vi "Autonomous Independent.vi"   [LabVIEW 2017]
doc: "This VI is called when autonomous begins, and will automatically be terminated when autonomous ends. You can carry out timed or sensor driven robot movement independently without needing to return to the caller."
uses:
  <vilib>/Rock Robotics/WPI/SafetyOutput/WPI_SafetyOutputConfigMenu.ctl
  <vilib>/Rock Robotics/Network Tables/NT Read String.vi
  <vilib>/Rock Robotics/Network Tables/NT Read Number.vi
  <vilib>/Rock Robotics/WPI/Utilities/WPI_GetSetVariantRefNum.vi
  <vilib>/Rock Robotics/WPI/RobotDrive/WPI_RobotDriveArcadeDrive_Standard(NoSaturation).vi
panel:
  # "Be sure to right-click and choose Data Operations>>Make Current Value default if you want to save the array values with the VI"
types:
  T1 = typedef "WPI_SafetyOutputConfigMenu.ctl" = enum16{"Enable", "Disable"}
  T2 = typedef "WPI_RobotDriveDevRef.ctl" = cluster{"DevStatus":errorcluster, "Motors[]":T3[], "Square Inputs":bool, "Max Output":dbl}
  T3 = typedef "WPI_MotorControlDeviceRef.ctl" = cluster{"DeviceStatus":errorcluster, "Type":T4, "PWM":cluster{"PWM Channel":T5, "DeadBand":T6}, "CAN":cluster{"Device Number":u8, "SetOutput VI Ref":variant, "GetOutput VI Ref":variant, "Enable VI Ref":variant, "Disable VI Ref":variant, "Data":variant}, "Invert":bool, "DIO PWM":cluster{"PWM \"Enable\" Channel":T5, "DIOChannel":T7, "PWM Rate":dbl}}
  T4 = typedef "WPI_MotorControlType.ctl" = enum16{"PWM", "CAN", "DIO PWM"}
  T5 = typedef "FPGA_DIOPWMChannel.ctl" = enum8{"PWM 0", "PWM 1", "PWM 2", "PWM 3", "PWM 4", "PWM 5", "PWM 6", "PWM 7", "PWM 8", "PWM 9", "PWM MXP 0", "PWM MXP 1", "PWM MXP 2", "PWM MXP 3", "PWM MXP 4", "PWM MXP 5", "PWM MXP 6", "PWM MXP 7", "PWM MXP 8", "PWM MXP 9", "Invalid"}
  T6 = typedef "WPI_PWMDeadband.ctl" = cluster{"Name":string, "maxPositivePwm":i32, "minPositivePwm":i32, "centerPwm":i32, "maxNegativePwm":i32, "minNegativePwm":i32, "angularRange":u16}
  T7 = typedef "FPGA_DIOChannel.ctl" = enum8{"DIO 0", "DIO 1", "DIO 2", "DIO 3", "DIO 4", "DIO 5", "DIO 6", "DIO 7", "DIO 8", "DIO 9", "DIO MXP 0", "DIO MXP 1", "DIO MXP 2", "DIO MXP 3", "DIO MXP 4", "DIO MXP 5", "DIO MXP 6", "DIO MXP 7", "DIO MXP 8", "DIO MXP 9", "DIO MXP 10", "DIO MXP 11", "DIO MXP 12", "DIO MXP 13", "DIO MXP 14", "DIO MXP 15", "SPI Port CS1", "SPI Port CS2", "SPI Port CS3", "SPI Port MISO", "SPI Port MOSI", "Invalid"}
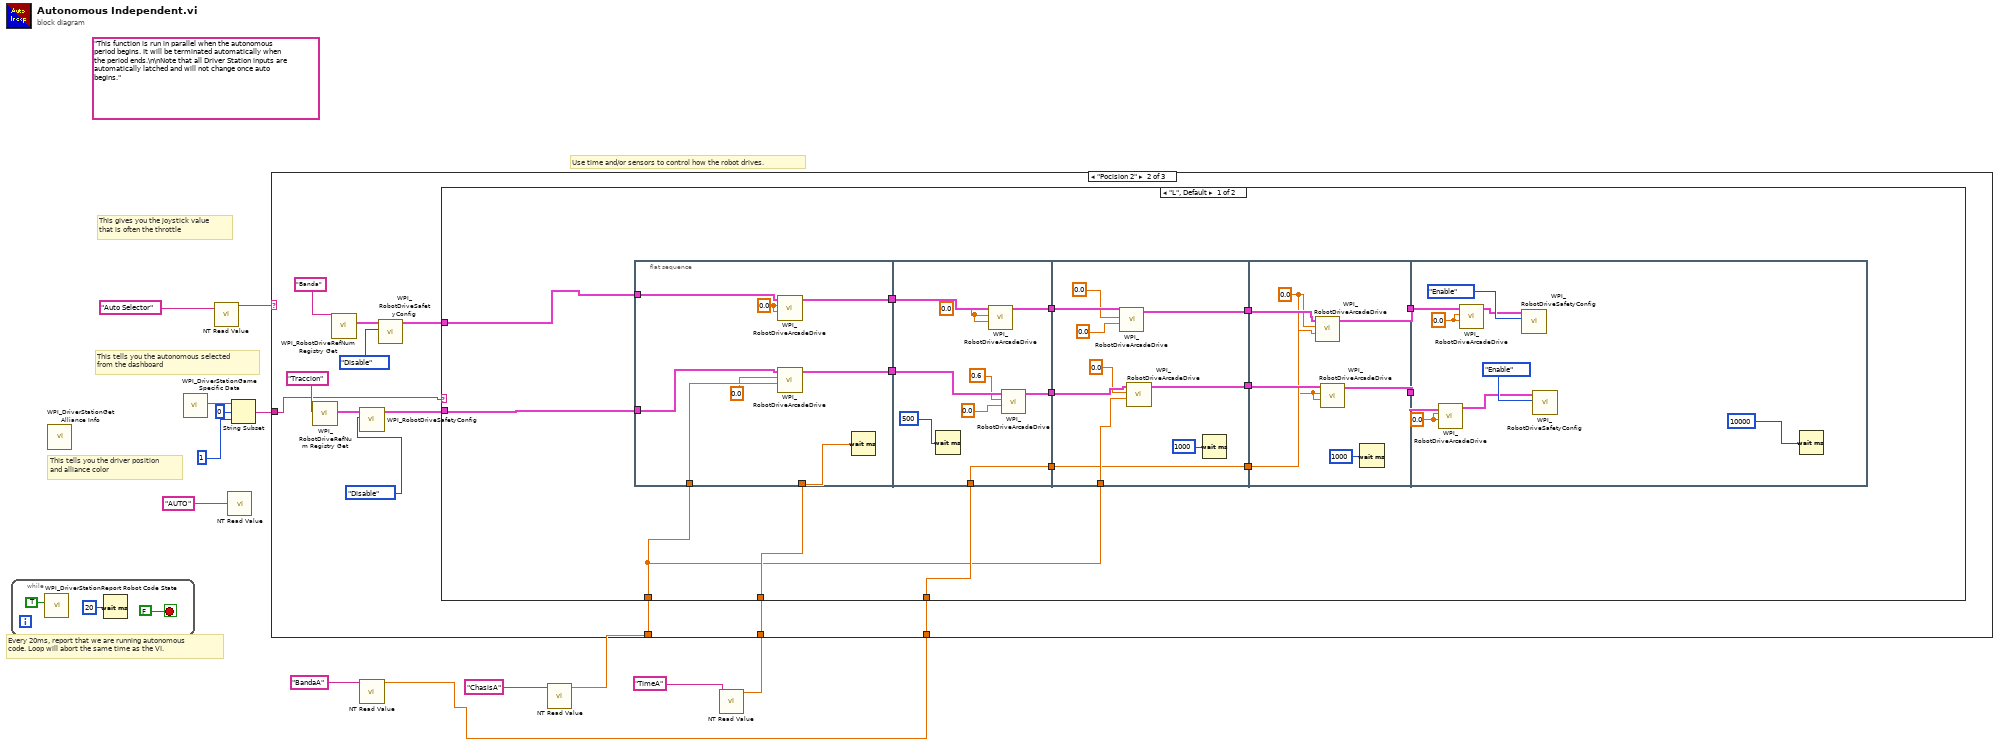
[diagram p0: block diagram]
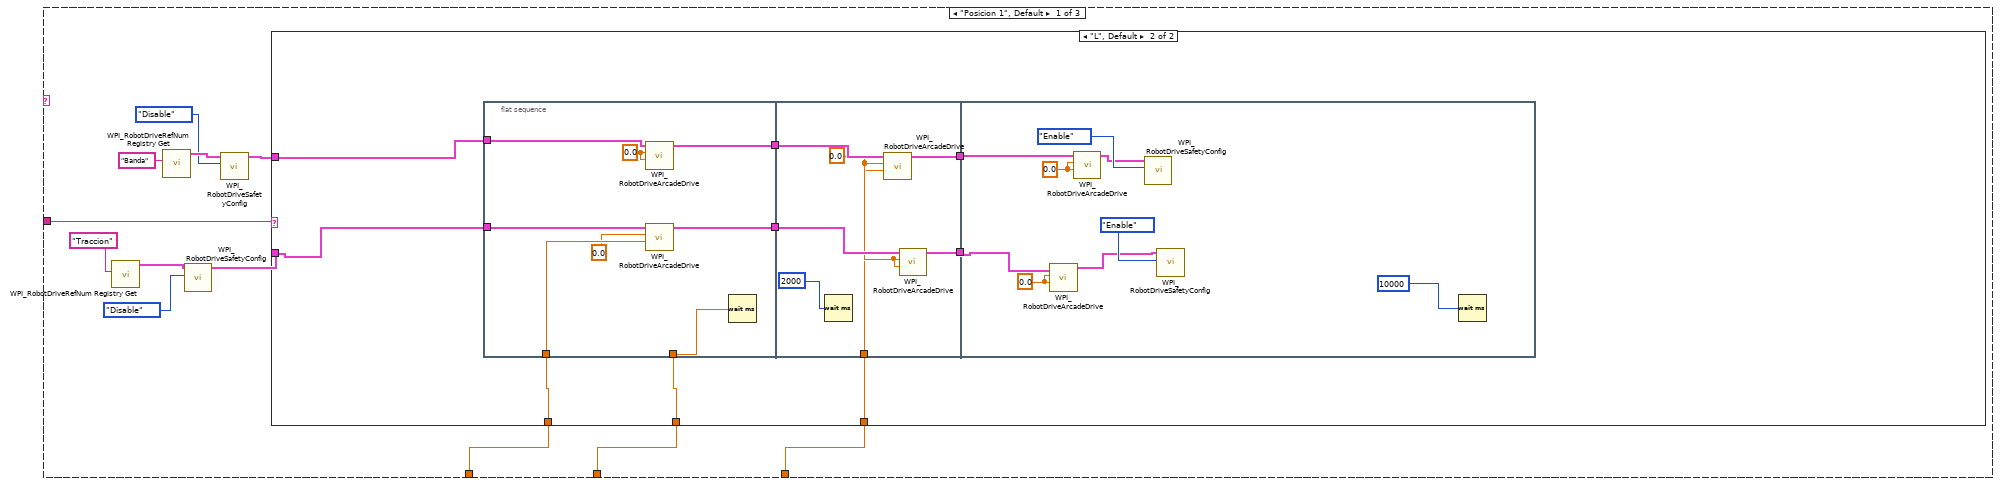
[diagram p2: hidden frame]
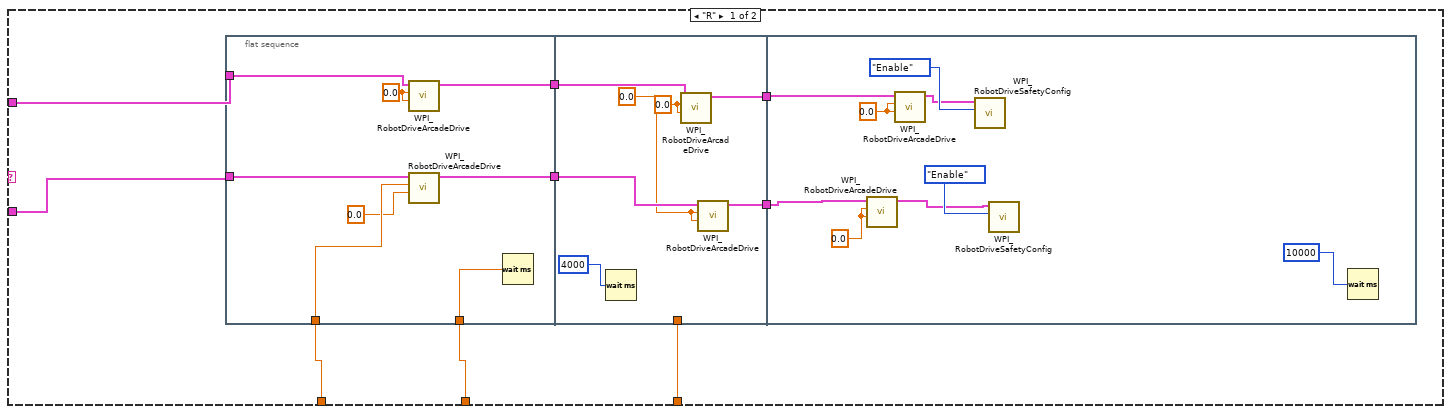
[diagram p3: hidden frame]
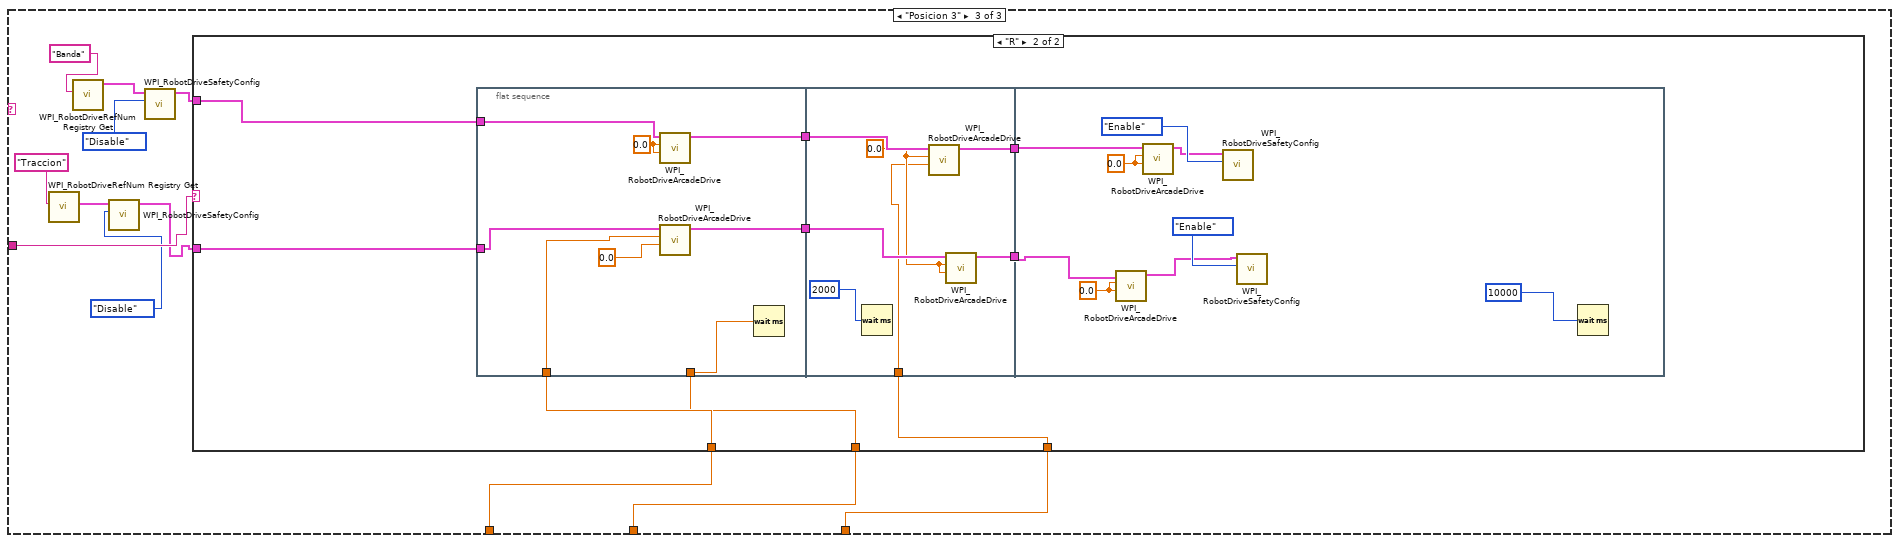
[diagram p5: hidden frame]
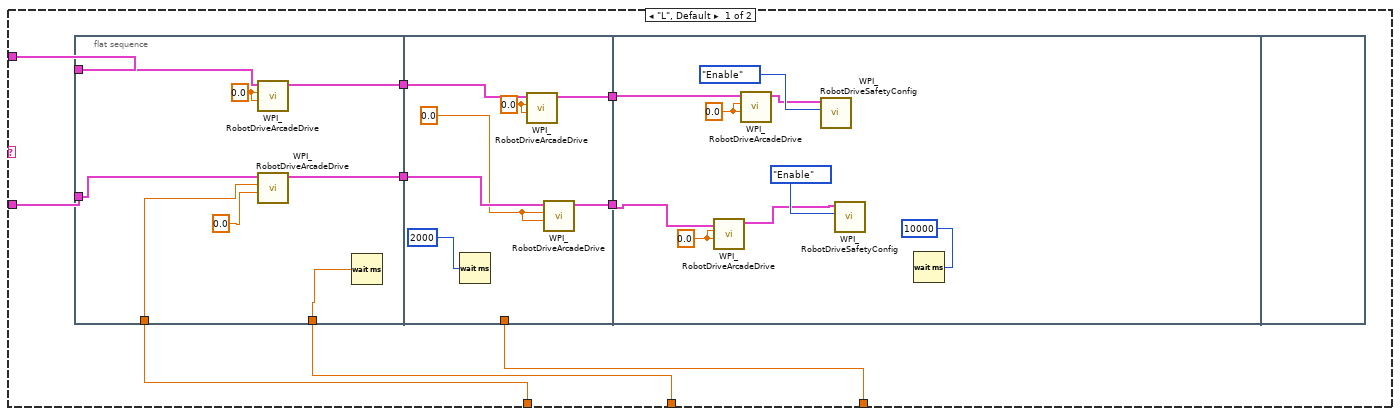
[diagram p6: hidden frame]
diagram:
  (unwired) "This function is run in parallel when the autonomous period begins. It will be terminated automatically when the period ends.\n\nNote that all Driver Station inputs are automatically latched and will not change once auto begins."
  # "This tells you the autonomous selected\nfrom the dashboard"
  # "Every 20ms, report that we are running autonomous\ncode. Loop will abort the same time as the VI."
  # "This gives you the joystick value\nthat is often the throttle"
  # "Use time and/or sensors to control how the robot drives."
  # "This tells you the driver position\nand alliance color"
  n1 = while {
    stop <- FALSE stop-if-true
    n2 = call <vilib>:"WPI_DriverStationReport Robot Code State.vi"("Autonomous"=TRUE) -> ()  [unwired: 10 in, 1 out]
    n3 = Wait (ms)(milliseconds to wait=u32 20) -> ()  [unwired: 1 out]
  }
  n4 = call <vilib>:"WPI_DriverStationGet Alliance Info.vi"() -> ()  [unwired: 12 out]
  n5 = call <vilib>:"WPI_DriverStationGame Specific Data.vi"() -> ("Game Specific Data"=w12:string)  [unwired: 11 in]
  n6 = call-poly <vilib>:"NT Read Value.vi"("Name"="Auto Selector") -> ("String"=w10:string)  [unwired: 9 in, 1 out]
  n7 = call-poly <vilib>:"NT Read Value.vi"("Name"="AUTO") -> ()  [unwired: 9 in, 2 out]
  n8 = String Subset(string=w12, offset (0)=0, length (rest)=1 ("length (rest)")) -> (substring=w1:string)
  n9 = call-poly <vilib>:"NT Read Value.vi"("Name"="BandaA") -> ("Numeric"=w2:dbl)  [unwired: 9 in, 1 out]
  n10 = call-poly <vilib>:"NT Read Value.vi"("Name"="ChasisA") -> ("Numeric"=w5:dbl)  [unwired: 9 in, 1 out]
  n11 = call-poly <vilib>:"NT Read Value.vi"("Name"="TimeA") -> ("Numeric"=w7:dbl)  [unwired: 9 in, 1 out]
  n12 = case shown="\"Pocision 2\"" w10 {
    tunnel: w1 -> [w28 w100 w175]
    tunnel: w7 -> [w27 w95 w167]
    tunnel: w5 -> [w26 w96 w168]
    tunnel: w2 -> [w25 w97 w166]
    frame "Posicion 1", Default {
      n13 = call <vilib>:"WPI_RobotDriveRefNum Registry Get.vi"("refnum name"="Traccion") -> ("RobotDriveDevRef"=w19:T2)  [unwired: 9 in, 1 out]
      n14 = call <vilib>:"WPI_RobotDriveRefNum Registry Get.vi"("refnum name"="Banda") -> ("RobotDriveDevRef"=w24:T2)  [unwired: 9 in, 1 out]
      n15 = call <vilib>:"WPI_RobotDriveSafetyConfig.vi"("mode"=WPI_SafetyOutputConfigMenu."Disable", "RobotDriveDevRef"=w19) -> ("RobotDriveDevRef"=w18:T2)  [unwired: 8 in, 1 out]
      n16 = call <vilib>:"WPI_RobotDriveSafetyConfig.vi"("mode"=WPI_SafetyOutputConfigMenu."Disable", "RobotDriveDevRef"=w24) -> ("RobotDriveDevRef"=w21:T2)  [unwired: 8 in, 1 out]
      n17 = case shown="\"L\", Default" w28 {
        tunnel: w27 -> [w37 w64]
        tunnel: w26 -> [w36 w63]
        tunnel: w25 -> [w33 w62]
        tunnel: w21 -> [w30 w66]
        tunnel: w18 -> [w29 w65]
        frame "R" {
          n18 = flat-sequence {
            tunnel: w37 -> [w45]
            tunnel: w36 -> [w39]
            tunnel: [w43] -> w35
            tunnel: [w42] -> w34
            tunnel: w30 -> [w41]
            tunnel: w29 -> [w40]
            tunnel: w35 -> [w52]
            tunnel: w34 -> [w51]
            tunnel: w33 -> [_]
            tunnel: [w49] -> w32
            tunnel: [w48] -> w31
            tunnel: w32 -> [w59]
            tunnel: w31 -> [w57]
            frame #0 {
              w44 = 0.0 ("X axis value")
              n19 = call-poly <vilib>:"WPI_RobotDriveArcadeDrive.vi"("Y axis value"=w44, "X axis value"=w44, "RobotDriveDevRef"=w41) -> ("RobotDriveDevRef"=w42:T2)  [unwired: 6 in, 2 out]
              n20 = call-poly <vilib>:"WPI_RobotDriveArcadeDrive.vi"("Y axis value"=0.0, "X axis value"=w39, "RobotDriveDevRef"=w40) -> ("RobotDriveDevRef"=w43:T2)  [unwired: 6 in, 2 out]
              n21 = Wait (ms)(milliseconds to wait=w45) -> ()  [unwired: 1 out]
            }
            frame #1 {
              w46 = 0.0 ("X axis value")
              w47 = 0.0 ("X axis value")
              n22 = Wait (ms)(milliseconds to wait=u32 4000) -> ()  [unwired: 1 out]
              n23 = call-poly <vilib>:"WPI_RobotDriveArcadeDrive.vi"("Y axis value"=w46, "X axis value"=w46, "RobotDriveDevRef"=w51) -> ("RobotDriveDevRef"=w49:T2)  [unwired: 6 in, 2 out]
              n24 = call-poly <vilib>:"WPI_RobotDriveArcadeDrive.vi"("Y axis value"=w47, "X axis value"=w47, "RobotDriveDevRef"=w52) -> ("RobotDriveDevRef"=w48:T2)  [unwired: 6 in, 2 out]
            }
            frame #2 {
              w55 = 0.0 ("Y axis value")
              w53 = 0.0 ("Y axis value")
              n25 = call-poly <vilib>:"WPI_RobotDriveArcadeDrive.vi"("Y axis value"=w53, "X axis value"=w53, "RobotDriveDevRef"=w57) -> ("RobotDriveDevRef"=w56:T2)  [unwired: 6 in, 2 out]
              n26 = call-poly <vilib>:"WPI_RobotDriveArcadeDrive.vi"("Y axis value"=w55, "X axis value"=w55, "RobotDriveDevRef"=w59) -> ("RobotDriveDevRef"=w58:T2)  [unwired: 6 in, 2 out]
              n27 = call <vilib>:"WPI_RobotDriveSafetyConfig.vi"("mode"=WPI_SafetyOutputConfigMenu."Enable", "RobotDriveDevRef"=w58) -> ()  [unwired: 8 in, 2 out]
              n28 = call <vilib>:"WPI_RobotDriveSafetyConfig.vi"("mode"=WPI_SafetyOutputConfigMenu."Enable", "RobotDriveDevRef"=w56) -> ()  [unwired: 8 in, 2 out]
              n29 = Wait (ms)(milliseconds to wait=u32 10000) -> ()  [unwired: 1 out]
            }
          }
        }
        frame "L", Default {
          n30 = flat-sequence {
            tunnel: [w77] -> w70
            tunnel: [w76] -> w69
            tunnel: w66 -> [w75]
            tunnel: w65 -> [w74]
            tunnel: w64 -> [w73]
            tunnel: w63 -> [w72]
            tunnel: w70 -> [w85]
            tunnel: w69 -> [w84]
            tunnel: [w82] -> w68
            tunnel: [w81] -> w67
            tunnel: w62 -> [w79]
            tunnel: w68 -> [w92]
            tunnel: w67 -> [w90]
            frame #0 {
              w78 = 0.0 ("X axis value")
              n31 = call-poly <vilib>:"WPI_RobotDriveArcadeDrive.vi"("Y axis value"=w78, "X axis value"=w78, "RobotDriveDevRef"=w75) -> ("RobotDriveDevRef"=w76:T2)  [unwired: 6 in, 2 out]
              n32 = call-poly <vilib>:"WPI_RobotDriveArcadeDrive.vi"("Y axis value"=w72, "X axis value"=0.0 ("Y axis value"), "RobotDriveDevRef"=w74) -> ("RobotDriveDevRef"=w77:T2)  [unwired: 6 in, 2 out]
              n33 = Wait (ms)(milliseconds to wait=w73) -> ()  [unwired: 1 out]
            }
            frame #1 {
              w80 = 0.0 ("X axis value")
              n34 = Wait (ms)(milliseconds to wait=u32 2000) -> ()  [unwired: 1 out]
              n35 = call-poly <vilib>:"WPI_RobotDriveArcadeDrive.vi"("Y axis value"=w79, "X axis value"=w80, "RobotDriveDevRef"=w84) -> ("RobotDriveDevRef"=w82:T2)  [unwired: 6 in, 2 out]
              n36 = call-poly <vilib>:"WPI_RobotDriveArcadeDrive.vi"("Y axis value"=w80, "X axis value"=w80, "RobotDriveDevRef"=w85) -> ("RobotDriveDevRef"=w81:T2)  [unwired: 6 in, 2 out]
            }
            frame #2 {
              w88 = 0.0 ("Y axis value")
              w86 = 0.0 ("Y axis value")
              n37 = call-poly <vilib>:"WPI_RobotDriveArcadeDrive.vi"("Y axis value"=w86, "X axis value"=w86, "RobotDriveDevRef"=w90) -> ("RobotDriveDevRef"=w89:T2)  [unwired: 6 in, 2 out]
              n38 = call-poly <vilib>:"WPI_RobotDriveArcadeDrive.vi"("Y axis value"=w88, "X axis value"=w88, "RobotDriveDevRef"=w92) -> ("RobotDriveDevRef"=w91:T2)  [unwired: 6 in, 2 out]
              n39 = call <vilib>:"WPI_RobotDriveSafetyConfig.vi"("mode"=WPI_SafetyOutputConfigMenu."Enable", "RobotDriveDevRef"=w91) -> ()  [unwired: 8 in, 2 out]
              n40 = call <vilib>:"WPI_RobotDriveSafetyConfig.vi"("mode"=WPI_SafetyOutputConfigMenu."Enable", "RobotDriveDevRef"=w89) -> ()  [unwired: 8 in, 2 out]
              n41 = Wait (ms)(milliseconds to wait=u32 10000) -> ()  [unwired: 1 out]
            }
          }
        }
      }
    }
    frame "Pocision 2" {
      n42 = call <vilib>:"WPI_RobotDriveRefNum Registry Get.vi"("refnum name"="Traccion") -> ("RobotDriveDevRef"=w106:T2)  [unwired: 9 in, 1 out]
      n43 = call <vilib>:"WPI_RobotDriveRefNum Registry Get.vi"("refnum name"="Banda") -> ("RobotDriveDevRef"=w102:T2)  [unwired: 9 in, 1 out]
      n44 = call <vilib>:"WPI_RobotDriveSafetyConfig.vi"("mode"=WPI_SafetyOutputConfigMenu."Disable", "RobotDriveDevRef"=w106) -> ("RobotDriveDevRef"=w98:T2)  [unwired: 8 in, 1 out]
      n45 = call <vilib>:"WPI_RobotDriveSafetyConfig.vi"("mode"=WPI_SafetyOutputConfigMenu."Disable", "RobotDriveDevRef"=w102) -> ("RobotDriveDevRef"=w99:T2)  [unwired: 8 in, 1 out]
      n46 = case shown="\"L\", Default" w100 {
        tunnel: w99 -> [w119 _]
        tunnel: w98 -> [w118 _]
        tunnel: w97 -> [w117 _]
        tunnel: w96 -> [w109 _]
        tunnel: w95 -> [w116 _]
        frame "L", Default {
          n47 = flat-sequence {
            tunnel: [w128] -> w121
            tunnel: [w127] -> w120
            tunnel: w119 -> [w126]
            tunnel: w116 -> [w125]
            tunnel: w109 -> [w124]
            tunnel: w118 -> [w122]
            tunnel: w121 -> [w138]
            tunnel: w120 -> [w137]
            tunnel: [w135] -> w115
            tunnel: [w134] -> w114
            tunnel: w117 -> [w130]
            tunnel: [w130] -> w107
            tunnel: w115 -> [w147]
            tunnel: w114 -> [w148]
            tunnel: [w143] -> w111
            tunnel: [w142] -> w110
            tunnel: w109 -> [w141]
            tunnel: [w140] -> w108
            tunnel: w107 -> [w140]
            tunnel: [w152] -> w113
            tunnel: [w153] -> w112
            tunnel: w111 -> [w155]
            tunnel: w110 -> [w154]
            tunnel: w108 -> [w151]
            tunnel: w113 -> [w162]
            tunnel: w112 -> [w160]
            frame #0 {
              w129 = 0.0 ("X axis value")
              n48 = call-poly <vilib>:"WPI_RobotDriveArcadeDrive.vi"("Y axis value"=w129, "X axis value"=w129, "RobotDriveDevRef"=w126) -> ("RobotDriveDevRef"=w127:T2)  [unwired: 6 in, 2 out]
              n49 = call-poly <vilib>:"WPI_RobotDriveArcadeDrive.vi"("Y axis value"=w124, "X axis value"=0.0 ("Y axis value"), "RobotDriveDevRef"=w122) -> ("RobotDriveDevRef"=w128:T2)  [unwired: 6 in, 2 out]
              n50 = Wait (ms)(milliseconds to wait=w125) -> ()  [unwired: 1 out]
            }
            frame #1 {
              w133 = 0.0 ("X axis value")
              n51 = Wait (ms)(milliseconds to wait=u32 500) -> ()  [unwired: 1 out]
              n52 = call-poly <vilib>:"WPI_RobotDriveArcadeDrive.vi"("Y axis value"=w133, "X axis value"=w133, "RobotDriveDevRef"=w137) -> ("RobotDriveDevRef"=w135:T2)  [unwired: 6 in, 2 out]
              n53 = call-poly <vilib>:"WPI_RobotDriveArcadeDrive.vi"("Y axis value"=0.0, "X axis value"=0.6, "RobotDriveDevRef"=w138) -> ("RobotDriveDevRef"=w134:T2)  [unwired: 6 in, 2 out]
            }
            frame #2 {
              n54 = call-poly <vilib>:"WPI_RobotDriveArcadeDrive.vi"("Y axis value"=0.0, "X axis value"=0.0, "RobotDriveDevRef"=w147) -> ("RobotDriveDevRef"=w143:T2)  [unwired: 6 in, 2 out]
              n55 = call-poly <vilib>:"WPI_RobotDriveArcadeDrive.vi"("Y axis value"=w141, "X axis value"=0.0, "RobotDriveDevRef"=w148) -> ("RobotDriveDevRef"=w142:T2)  [unwired: 6 in, 2 out]
              n56 = Wait (ms)(milliseconds to wait=u32 1000) -> ()  [unwired: 1 out]
            }
            frame #3 {
              w150 = 0.0 ("X axis value")
              n57 = call-poly <vilib>:"WPI_RobotDriveArcadeDrive.vi"("Y axis value"=w151, "X axis value"=w150, "RobotDriveDevRef"=w155) -> ("RobotDriveDevRef"=w152:T2)  [unwired: 6 in, 2 out]
              n58 = call-poly <vilib>:"WPI_RobotDriveArcadeDrive.vi"("Y axis value"=w150, "X axis value"=w150, "RobotDriveDevRef"=w154) -> ("RobotDriveDevRef"=w153:T2)  [unwired: 6 in, 2 out]
              n59 = Wait (ms)(milliseconds to wait=u32 1000) -> ()  [unwired: 1 out]
            }
            frame #4 {
              w158 = 0.0 ("Y axis value")
              w156 = 0.0 ("Y axis value")
              n60 = call-poly <vilib>:"WPI_RobotDriveArcadeDrive.vi"("Y axis value"=w156, "X axis value"=w156, "RobotDriveDevRef"=w160) -> ("RobotDriveDevRef"=w159:T2)  [unwired: 6 in, 2 out]
              n61 = call-poly <vilib>:"WPI_RobotDriveArcadeDrive.vi"("Y axis value"=w158, "X axis value"=w158, "RobotDriveDevRef"=w162) -> ("RobotDriveDevRef"=w161:T2)  [unwired: 6 in, 2 out]
              n62 = call <vilib>:"WPI_RobotDriveSafetyConfig.vi"("mode"=WPI_SafetyOutputConfigMenu."Enable", "RobotDriveDevRef"=w161) -> ()  [unwired: 8 in, 2 out]
              n63 = call <vilib>:"WPI_RobotDriveSafetyConfig.vi"("mode"=WPI_SafetyOutputConfigMenu."Enable", "RobotDriveDevRef"=w159) -> ()  [unwired: 8 in, 2 out]
              n64 = Wait (ms)(milliseconds to wait=u32 10000) -> ()  [unwired: 1 out]
            }
          }
        }
        frame "B" {
        }
      }
    }
    frame "Posicion 3" {
      n65 = call <vilib>:"WPI_RobotDriveRefNum Registry Get.vi"("refnum name"="Traccion") -> ("RobotDriveDevRef"=w176:T2)  [unwired: 9 in, 1 out]
      n66 = call <vilib>:"WPI_RobotDriveRefNum Registry Get.vi"("refnum name"="Banda") -> ("RobotDriveDevRef"=w169:T2)  [unwired: 9 in, 1 out]
      n67 = call <vilib>:"WPI_RobotDriveSafetyConfig.vi"("mode"=WPI_SafetyOutputConfigMenu."Disable", "RobotDriveDevRef"=w176) -> ("RobotDriveDevRef"=w173:T2)  [unwired: 8 in, 1 out]
      n68 = call <vilib>:"WPI_RobotDriveSafetyConfig.vi"("mode"=WPI_SafetyOutputConfigMenu."Disable", "RobotDriveDevRef"=w169) -> ("RobotDriveDevRef"=w172:T2)  [unwired: 8 in, 1 out]
      n69 = case shown="\"R\"" w175 {
        tunnel: w173 -> [w180 w214]
        tunnel: w172 -> [w181 w213]
        tunnel: w168 -> [w178 w212]
        tunnel: w167 -> [w179 w211]
        tunnel: w166 -> [w177 w210]
        frame "L", Default {
          n70 = flat-sequence {
            tunnel: [w192] -> w185
            tunnel: [w191] -> w184
            tunnel: w178 -> [w187]
            tunnel: w180 -> [w190]
            tunnel: w181 -> [w189]
            tunnel: w179 -> [w188]
            tunnel: w185 -> [w200]
            tunnel: w184 -> [w199]
            tunnel: [w197] -> w183
            tunnel: [w196] -> w182
            tunnel: w177 -> [_]
            tunnel: w183 -> [w207]
            tunnel: w182 -> [w205]
            frame #0 {
              w193 = 0.0 ("X axis value")
              n71 = call-poly <vilib>:"WPI_RobotDriveArcadeDrive.vi"("Y axis value"=w193, "X axis value"=w193, "RobotDriveDevRef"=w189) -> ("RobotDriveDevRef"=w191:T2)  [unwired: 6 in, 2 out]
              n72 = call-poly <vilib>:"WPI_RobotDriveArcadeDrive.vi"("Y axis value"=0.0, "X axis value"=w187, "RobotDriveDevRef"=w190) -> ("RobotDriveDevRef"=w192:T2)  [unwired: 6 in, 2 out]
              n73 = Wait (ms)(milliseconds to wait=w188) -> ()  [unwired: 1 out]
            }
            frame #1 {
              w194 = 0.0 ("X axis value")
              w195 = 0.0 ("X axis value")
              n74 = Wait (ms)(milliseconds to wait=u32 2000) -> ()  [unwired: 1 out]
              n75 = call-poly <vilib>:"WPI_RobotDriveArcadeDrive.vi"("Y axis value"=w194, "X axis value"=w194, "RobotDriveDevRef"=w199) -> ("RobotDriveDevRef"=w197:T2)  [unwired: 6 in, 2 out]
              n76 = call-poly <vilib>:"WPI_RobotDriveArcadeDrive.vi"("Y axis value"=w195, "X axis value"=w195, "RobotDriveDevRef"=w200) -> ("RobotDriveDevRef"=w196:T2)  [unwired: 6 in, 2 out]
            }
            frame #2 {
              w203 = 0.0 ("Y axis value")
              w201 = 0.0 ("Y axis value")
              n77 = call-poly <vilib>:"WPI_RobotDriveArcadeDrive.vi"("Y axis value"=w201, "X axis value"=w201, "RobotDriveDevRef"=w205) -> ("RobotDriveDevRef"=w204:T2)  [unwired: 6 in, 2 out]
              n78 = call-poly <vilib>:"WPI_RobotDriveArcadeDrive.vi"("Y axis value"=w203, "X axis value"=w203, "RobotDriveDevRef"=w207) -> ("RobotDriveDevRef"=w206:T2)  [unwired: 6 in, 2 out]
              n79 = call <vilib>:"WPI_RobotDriveSafetyConfig.vi"("mode"=WPI_SafetyOutputConfigMenu."Enable", "RobotDriveDevRef"=w206) -> ()  [unwired: 8 in, 2 out]
              n80 = call <vilib>:"WPI_RobotDriveSafetyConfig.vi"("mode"=WPI_SafetyOutputConfigMenu."Enable", "RobotDriveDevRef"=w204) -> ()  [unwired: 8 in, 2 out]
              n81 = Wait (ms)(milliseconds to wait=u32 10000) -> ()  [unwired: 1 out]
            }
            frame #3 {
            }
          }
        }
        frame "R" {
          n82 = flat-sequence {
            tunnel: [w225] -> w218
            tunnel: [w224] -> w217
            tunnel: w211 -> [w223]
            tunnel: w212 -> [w220]
            tunnel: w214 -> [w222]
            tunnel: w213 -> [w221]
            tunnel: w218 -> [w233]
            tunnel: w217 -> [w232]
            tunnel: [w230] -> w216
            tunnel: [w229] -> w215
            tunnel: w210 -> [w227]
            tunnel: w216 -> [w240]
            tunnel: w215 -> [w238]
            frame #0 {
              w226 = 0.0 ("X axis value")
              n83 = call-poly <vilib>:"WPI_RobotDriveArcadeDrive.vi"("Y axis value"=w226, "X axis value"=w226, "RobotDriveDevRef"=w221) -> ("RobotDriveDevRef"=w224:T2)  [unwired: 6 in, 2 out]
              n84 = call-poly <vilib>:"WPI_RobotDriveArcadeDrive.vi"("Y axis value"=0.0, "X axis value"=w220, "RobotDriveDevRef"=w222) -> ("RobotDriveDevRef"=w225:T2)  [unwired: 6 in, 2 out]
              n85 = Wait (ms)(milliseconds to wait=w223) -> ()  [unwired: 1 out]
            }
            frame #1 {
              w228 = 0.0 ("X axis value")
              n86 = Wait (ms)(milliseconds to wait=u32 2000) -> ()  [unwired: 1 out]
              n87 = call-poly <vilib>:"WPI_RobotDriveArcadeDrive.vi"("Y axis value"=w227, "X axis value"=w228, "RobotDriveDevRef"=w232) -> ("RobotDriveDevRef"=w230:T2)  [unwired: 6 in, 2 out]
              n88 = call-poly <vilib>:"WPI_RobotDriveArcadeDrive.vi"("Y axis value"=w228, "X axis value"=w228, "RobotDriveDevRef"=w233) -> ("RobotDriveDevRef"=w229:T2)  [unwired: 6 in, 2 out]
            }
            frame #2 {
              w236 = 0.0 ("Y axis value")
              w234 = 0.0 ("Y axis value")
              n89 = call-poly <vilib>:"WPI_RobotDriveArcadeDrive.vi"("Y axis value"=w234, "X axis value"=w234, "RobotDriveDevRef"=w238) -> ("RobotDriveDevRef"=w237:T2)  [unwired: 6 in, 2 out]
              n90 = call-poly <vilib>:"WPI_RobotDriveArcadeDrive.vi"("Y axis value"=w236, "X axis value"=w236, "RobotDriveDevRef"=w240) -> ("RobotDriveDevRef"=w239:T2)  [unwired: 6 in, 2 out]
              n91 = call <vilib>:"WPI_RobotDriveSafetyConfig.vi"("mode"=WPI_SafetyOutputConfigMenu."Enable", "RobotDriveDevRef"=w239) -> ()  [unwired: 8 in, 2 out]
              n92 = call <vilib>:"WPI_RobotDriveSafetyConfig.vi"("mode"=WPI_SafetyOutputConfigMenu."Enable", "RobotDriveDevRef"=w237) -> ()  [unwired: 8 in, 2 out]
              n93 = Wait (ms)(milliseconds to wait=u32 10000) -> ()  [unwired: 1 out]
            }
          }
        }
      }
    }
  }
